vi "Lab Panel V5.24.1.vi"() -> ()   [LabVIEW 2013] (continued)
                          tunnel: [errorcluster {"status"=FALSE, "code"=0, "source"=""} ("error out") w884] -> w871
                          tunnel: w870 -> [_ w883]
                          tunnel: w869 -> [_ w882]
                          tunnel: w868 -> [_ w881]
                          tunnel: w867 -> [_ w880]
                          tunnel: w865 -> [_ w879]
                          frame False {
                            w877 = FALSE
                            n582 = local write "RUN LAB01-2"(w877) -> ()
                            n583 = local write "run lab01-2"(w877) -> ()
                          }
                          frame True {
                            n584 = stacked-sequence {
                              seq-local: [w890 _ _ _ _] -> [_ w914 _ _ _]
                              tunnel: w889 -> [w895 _ _ _ _]
                              tunnel: w888 -> [w892 _ _ _ _]
                              tunnel: w887 -> [w905 _ _ _ _]
                              tunnel: w886 -> [w898 _ _ _ _]
                              tunnel: w885 -> [w893 _ _ _ _]
                              tunnel: [_ w909 _ _ _] -> w884
                              tunnel: w883 -> [_ _ _ w936 _]
                              tunnel: w882 -> [_ _ _ w935 _]
                              tunnel: w881 -> [_ _ _ w934 _]
                              tunnel: w880 -> [_ _ _ _ _]
                              tunnel: w879 -> [_ _ _ _ w949]
                              frame #0 {
                                w891 = "\\"
                                n585 = local read "SET LAB01-2"() -> (w900:T5)
                                n586 = case shown="\"CYCLE TEST\"" w905 {
                                tunnel: ["L01-2-CHART TEST-" "L01-2-CYCLE TEST-" "L01-2-T-RISE TEST-"] -> w901
                                frame "CHART TEST", Default {
                                }
                                frame "CYCLE TEST" {
                                }
                                frame "T-RISE TEST" {
                                }
                                }
                                n587 = Unbundle(w900) -> ("DESCRIPTION"=w899:string)  [unwired: 4 out]
                                n588 = Concatenate Strings(w895, "\\", w893, w891, w892, w891) -> (w902:string)
                                n589 = String To Path(string=w902) -> (path=w904:path)
                                n590 = Concatenate Strings(w902, w901, w899, "-", w898, ".tdms") -> (w890:string)
                                n591 = Create Folder(path (use dialog)=w904) -> (error out=w903:errorcluster)  [unwired: 2 in, 2 out]
                                n592 = call <vilib>:"Clear Errors.vi"("error in (no error)"=w903) -> ()  [unwired: 6 in, 1 out]
                                n593 = global write "Global 1.vi" "LAB01-2 FILE"(w890) -> ()
                              }
                              frame #1 {
                                (unwired) FALSE
                                n594 = String To Path(string=w914) -> (path=w910:path)
                                n595 = TDMS Open(6:FALSE, 10:T21."create or replace" ("operation (0:open)"), 11:w910) -> (0:w909:errorcluster, 3:→"TDMS LAB01-2":refnum<k34>)  [unwired: 4 in]
                              }
                              frame #2 {
                                n596 = local read "SET LAB01-2"() -> (w920:T5)
                                n597 = local read "TDMS LAB01-2"() -> (w931:refnum<k34>)
                                n598 = Build Array("Testers Name", "Description", "Set Test Cycles", "T-Rise minutes", "T-Rise Deg C") -> (w921:string[])
                                n599 = Unbundle(w920) -> ("NAME"=w919:string, "DESCRIPTION"=w918:string, "CYCLES"=w917:dbl, "T-RISE mins"=w916:dbl, "T-RISE deg C"=w915:dbl)
                                n600 = Number To Decimal String(number=w917) -> (decimal integer string=w930:string)  [unwired: 1 in]
                                n601 = Number To Decimal String(number=w916) -> (decimal integer string=w929:string)  [unwired: 1 in]
                                n602 = Number To Decimal String(number=w915) -> (decimal integer string=w928:string)  [unwired: 1 in]
                                n603 = Build Array(w919, w918, w930, w929, w928) -> (w927:string[])
                                n604 = TDMS Set Properties(5:w927, 7:w921, 11:w931) -> ()  [unwired: 3 in, 4 out]
                              }
                              frame #3 {
                                n605 = local read "DISP LAB01-2"() -> (w933:T4)
                                n606 = Concatenate Strings("LAB01-2  ", w936) -> (w937:string)
                                n607 = Two Button Dialog(message=w937, 1:w934, 2:w935) -> (T button?=w939:bool)
                                n608 = case shown="True" w939 {
                                tunnel: w933 -> [w946 w947]
                                tunnel: [w946 w947] -> w943
                                tunnel: [w945 w948] -> w942
                                tunnel: [w944 w948] -> w941
                                frame False {
                                n609 = Unbundle(w946) -> ("CYCLE"=w945:dbl, "MINS"=w944:dbl)  [unwired: 1 out]
                                }
                                frame True {
                                w948 = 0.0
                                }
                                }
                                n610 = Bundle(cluster=w943, "CYCLE"=w942, "MINS"=w941, "STATUS"="RUN") -> (w932:T4)
                                n611 = local write "DISP LAB01-2"(w932) -> ()
                              }
                              frame #4 {
                                n612 = local read "TEMP START LAB01-2"() -> (w951:cluster{"TL":dbl, "TN":dbl})
                                n613 = Bundle(cluster=w951, "TL"=w949, "TN"=w949) -> (w950:cluster{"TL":dbl, "TN":dbl})
                                n614 = local write "TEMP START LAB01-2"(w950) -> ()
                              }
                            }
                          }
                        }
                      }
                    }
                  }
                }
              }
              event "RUN LAB02-1": Value Change {
                n615 = event-data() -> ("NewVal"=w957:bool)  [unwired: 1 in, 5 out]
                n616 = local read "SIG LAB02-1"() -> (w953:T2)
                n617 = case shown="True" w957 {
                  tunnel: w963 -> [_ w1001]
                  tunnel: w962 -> [_ w1000]
                  tunnel: w960 -> [w965 w999]
                  tunnel: w961 -> [_ w998]
                  tunnel: w959 -> [_ w997]
                  tunnel: [w964 w996] -> w958
                  tunnel: w956 -> [_ w995]
                  tunnel: w955 -> [_ w994]
                  tunnel: w954 -> [_ w993]
                  tunnel: w953 -> [_ w992]
                  tunnel: w952 -> [_ w991]
                  frame False {
                    # "stop test"
                    n618 = stacked-sequence {
                      tunnel: w965 -> [w974 _]
                      tunnel: [w966 _] -> w964
                      frame #0 {
                        n619 = local read "DISP LAB02-1"() -> (w973:T4)
                        n620 = Unbundle(w973) -> ("CYCLE"=w971:dbl, "MINS"=w972:dbl)  [unwired: 1 out]
                        n621 = case shown="\"CYCLE TEST\"" w974 {
                          tunnel: w972 -> [_ _ w981]
                          tunnel: w971 -> [w979 w980 _]
                          tunnel: [w979 w980 w981] -> w970
                          frame "CHART TEST", Default {
                          }
                          frame "CYCLE TEST" {
                          }
                          frame "T-RISE TEST" {
                          }
                        }
                        n622 = local read "TDMS LAB02-1"() -> (w978:refnum<k34>)
                        n623 = Build Array("STOPPED") -> (w975:string[])
                        n624 = Build Array(w970) -> (w969:dbl[])
                        n625 = TDMS Write(0:w978, 5:"TEST RESULT", 7:w975, 9:w969) -> (4:w967:refnum<k34>, 15:w968:errorcluster)  [unwired: 2 in, 2 out]
                        n626 = TDMS Close(8:w968, 11:w967) -> (0:w966:errorcluster)  [unwired: 1 out]
                      }
                      frame #1 {
                        n627 = local read "DISP LAB02-1"() -> (w985:T4)
                        n628 = stacked-sequence {
                          tunnel: "LAB02-1" -> [w987 w989]
                          frame #0 {
                            n629 = call "sub vi - defrag tdms v1.vi"("panel id"=w987) -> ("error out"=w986:errorcluster)  [unwired: 10 in]
                            n630 = local write "data file error"(w986) -> ()
                          }
                          frame #1 {
                            n631 = local write "RESULT LAB02-1"(FALSE) -> ()
                            n632 = call "Save data file (stop) v3.vi"("panel id"=w989) -> ("network file save error"=w988:errorcluster)  [unwired: 9 in, 1 out]
                            n633 = local write "data file error"(w988) -> ()
                          }
                        }
                        n634 = Bundle(cluster=w985, "STATUS"="STOP") -> (w983:T4)  [unwired: 2 in]
                        n635 = local write "DISP LAB02-1"(w983) -> ()
                      }
                    }
                  }
                  frame True {
                    n636 = stacked-sequence {
                      seq-local: [w1003 _] -> [_ w1007]
                      tunnel: w1001 -> [_ w1017]
                      tunnel: w1000 -> [_ w1016]
                      tunnel: w999 -> [_ w1015]
                      tunnel: w998 -> [_ w1014]
                      tunnel: w997 -> [_ w1013]
                      tunnel: [_ w1012] -> w996
                      tunnel: w995 -> [_ w1011]
                      tunnel: w994 -> [_ w1010]
                      tunnel: w993 -> [_ w1009]
                      tunnel: w992 -> [w1002 w1008]
                      tunnel: w991 -> [_ w1006]
                      frame #0 {
                        n637 = Unbundle(w1002) -> ("AMPS"=w1005:dbl)  [unwired: 4 out]
                        n638 = call "Check For Amps on v1.vi"("ID"="LAB02-1", "amps"=w1005) -> ("amps"=w1003:bool)  [unwired: 9 in]
                      }
                      frame #1 {
                        n639 = case shown="True" w1007 {
                          tunnel: w1017 -> [_ w1030]
                          tunnel: w1016 -> [_ w1029]
                          tunnel: w1015 -> [_ w1028]
                          tunnel: w1014 -> [_ w1027]
                          tunnel: w1013 -> [_ w1026]
                          tunnel: [errorcluster {"status"=FALSE, "code"=0, "source"=""} ("error out") w1025] -> w1012
                          tunnel: w1011 -> [_ w1024]
                          tunnel: w1010 -> [_ w1023]
                          tunnel: w1009 -> [_ w1022]
                          tunnel: w1008 -> [_ w1021]
                          tunnel: w1006 -> [_ w1020]
                          frame False {
                            w1019 = FALSE
                            n640 = local write "RUN LAB02-1"(w1019) -> ()
                            n641 = local write "run lab02-1"(w1019) -> ()
                          }
                          frame True {
                            n642 = stacked-sequence {
                              seq-local: [w1031 _ _ _ _] -> [_ w1055 _ _ _]
                              tunnel: w1030 -> [w1036 _ _ _ _]
                              tunnel: w1029 -> [w1033 _ _ _ _]
                              tunnel: w1028 -> [w1046 _ _ _ _]
                              tunnel: w1027 -> [w1039 _ _ _ _]
                              tunnel: w1026 -> [w1034 _ _ _ _]
                              tunnel: [_ w1050 _ _ _] -> w1025
                              tunnel: w1024 -> [_ _ _ w1076 _]
                              tunnel: w1023 -> [_ _ _ w1075 _]
                              tunnel: w1022 -> [_ _ _ w1074 _]
                              tunnel: w1021 -> [_ _ _ _ _]
                              tunnel: w1020 -> [_ _ _ _ w1090]
                              frame #0 {
                                w1032 = "\\"
                                n643 = local read "SET LAB02-1"() -> (w1041:T5)
                                n644 = case shown="\"CYCLE TEST\"" w1046 {
                                tunnel: ["L02-1-CHART TEST-" "L02-1-CYCLE TEST-" "L02-1-T-RISE TEST-"] -> w1042
                                frame "CHART TEST", Default {
                                }
                                frame "CYCLE TEST" {
                                }
                                frame "T-RISE TEST" {
                                }
                                }
                                n645 = Unbundle(w1041) -> ("DESCRIPTION"=w1040:string)  [unwired: 4 out]
                                n646 = Concatenate Strings(w1036, "\\", w1034, w1032, w1033, w1032) -> (w1043:string)
                                n647 = String To Path(string=w1043) -> (path=w1045:path)
                                n648 = Concatenate Strings(w1043, w1042, w1040, "-", w1039, ".tdms") -> (w1031:string)
                                n649 = Create Folder(path (use dialog)=w1045) -> (error out=w1044:errorcluster)  [unwired: 2 in, 2 out]
                                n650 = global write "Global 1.vi" "LAB02-1 FILE"(w1031) -> ()
                                n651 = call <vilib>:"Clear Errors.vi"("error in (no error)"=w1044) -> ()  [unwired: 6 in, 1 out]
                              }
                              frame #1 {
                                (unwired) FALSE
                                n652 = String To Path(string=w1055) -> (path=w1051:path)
                                n653 = TDMS Open(6:FALSE, 10:T21."create or replace" ("operation (0:open)"), 11:w1051) -> (0:w1050:errorcluster, 3:→"TDMS LAB02-1":refnum<k34>)  [unwired: 4 in]
                              }
                              frame #2 {
                                n654 = local read "SET LAB02-1"() -> (w1061:T5)
                                n655 = local read "TDMS LAB02-1"() -> (w1072:refnum<k34>)
                                n656 = Build Array("Testers Name", "Description", "Set Test Cycles", "T-Rise minutes", "T-Rise Deg C") -> (w1062:string[])
                                n657 = Unbundle(w1061) -> ("NAME"=w1060:string, "DESCRIPTION"=w1059:string, "CYCLES"=w1058:dbl, "T-RISE mins"=w1057:dbl, "T-RISE deg C"=w1056:dbl)
                                n658 = Number To Decimal String(number=w1058) -> (decimal integer string=w1071:string)  [unwired: 1 in]
                                n659 = Number To Decimal String(number=w1057) -> (decimal integer string=w1070:string)  [unwired: 1 in]
                                n660 = Number To Decimal String(number=w1056) -> (decimal integer string=w1069:string)  [unwired: 1 in]
                                n661 = Build Array(w1060, w1059, w1071, w1070, w1069) -> (w1068:string[])
                                n662 = TDMS Set Properties(5:w1068, 7:w1062, 11:w1072) -> ()  [unwired: 3 in, 4 out]
                              }
                              frame #3 {
                                n663 = local read "DISP LAB02-1"() -> (w1077:T4)
                                n664 = Concatenate Strings("LAB02-1  ", w1076) -> (w1078:string)
                                n665 = Two Button Dialog(message=w1078, 1:w1074, 2:w1075) -> (T button?=w1080:bool)
                                n666 = case shown="True" w1080 {
                                tunnel: w1077 -> [w1087 w1088]
                                tunnel: [w1087 w1088] -> w1084
                                tunnel: [w1086 w1089] -> w1083
                                tunnel: [w1085 w1089] -> w1082
                                frame False {
                                n667 = Unbundle(w1087) -> ("CYCLE"=w1086:dbl, "MINS"=w1085:dbl)  [unwired: 1 out]
                                }
                                frame True {
                                w1089 = 0.0
                                }
                                }
                                n668 = Bundle(cluster=w1084, "CYCLE"=w1083, "MINS"=w1082, "STATUS"="RUN") -> (w1073:T4)
                                n669 = local write "DISP LAB02-1"(w1073) -> ()
                              }
                              frame #4 {
                                n670 = local read "TEMP START LAB02-1"() -> (w1092:cluster{"TL":dbl, "TN":dbl})
                                n671 = Bundle(cluster=w1092, "TL"=w1090, "TN"=w1090) -> (w1091:cluster{"TL":dbl, "TN":dbl})
                                n672 = local write "TEMP START LAB02-1"(w1091) -> ()
                              }
                            }
                          }
                        }
                      }
                    }
                  }
                }
                n673 = local write "run lab02-1"(w957) -> ()
              }
              event "RUN LAB02-2": Value Change {
                n674 = event-data() -> ("NewVal"=w1097:bool)  [unwired: 1 in, 5 out]
                n675 = local write "run lab02-2"(w1097) -> ()
                n676 = case shown="True" w1097 {
                  tunnel: w1103 -> [_ w1141]
                  tunnel: w1102 -> [_ w1140]
                  tunnel: w1100 -> [w1105 w1139]
                  tunnel: w1101 -> [_ w1138]
                  tunnel: w1099 -> [_ w1137]
                  tunnel: [w1104 w1136] -> w1098
                  tunnel: w1096 -> [_ w1135]
                  tunnel: w1095 -> [_ w1134]
                  tunnel: w1094 -> [_ w1133]
                  tunnel: w1093 -> [_ w1131]
                  frame False {
                    # "stop test"
                    n677 = stacked-sequence {
                      tunnel: w1105 -> [w1114 _]
                      tunnel: [w1106 _] -> w1104
                      frame #0 {
                        n678 = local read "DISP LAB02-2"() -> (w1113:T4)
                        n679 = Unbundle(w1113) -> ("CYCLE"=w1111:dbl, "MINS"=w1112:dbl)  [unwired: 1 out]
                        n680 = case shown="\"CYCLE TEST\"" w1114 {
                          tunnel: w1112 -> [_ _ w1121]
                          tunnel: w1111 -> [w1119 w1120 _]
                          tunnel: [w1119 w1120 w1121] -> w1110
                          frame "CHART TEST", Default {
                          }
                          frame "CYCLE TEST" {
                          }
                          frame "T-RISE TEST" {
                          }
                        }
                        n681 = local read "TDMS LAB02-2"() -> (w1118:refnum<k34>)
                        n682 = Build Array("STOPPED") -> (w1115:string[])
                        n683 = Build Array(w1110) -> (w1109:dbl[])
                        n684 = TDMS Write(0:w1118, 5:"TEST RESULT", 7:w1115, 9:w1109) -> (4:w1107:refnum<k34>, 15:w1108:errorcluster)  [unwired: 2 in, 2 out]
                        n685 = TDMS Close(8:w1108, 11:w1107) -> (0:w1106:errorcluster)  [unwired: 1 out]
                      }
                      frame #1 {
                        n686 = local read "DISP LAB02-2"() -> (w1125:T4)
                        n687 = stacked-sequence {
                          tunnel: "LAB02-2" -> [w1127 w1129]
                          frame #0 {
                            n688 = call "sub vi - defrag tdms v1.vi"("panel id"=w1127) -> ("error out"=w1126:errorcluster)  [unwired: 10 in]
                            n689 = local write "data file error"(w1126) -> ()
                          }
                          frame #1 {
                            n690 = call "Save data file (stop) v3.vi"("panel id"=w1129) -> ("network file save error"=w1128:errorcluster)  [unwired: 9 in, 1 out]
                            n691 = local write "RESULT LAB02-2"(FALSE) -> ()
                            n692 = local write "data file error"(w1128) -> ()
                          }
                        }
                        n693 = Bundle(cluster=w1125, "STATUS"="STOP") -> (w1123:T4)  [unwired: 2 in]
                        n694 = local write "DISP LAB02-2"(w1123) -> ()
                      }
                    }
                  }
                  frame True {
                    n695 = local read "SIG LAB02-2"() -> (w1132:T2)
                    n696 = stacked-sequence {
                      seq-local: [w1143 _] -> [_ w1147]
                      tunnel: w1141 -> [_ w1157]
                      tunnel: w1140 -> [_ w1156]
                      tunnel: w1139 -> [_ w1155]
                      tunnel: w1138 -> [_ w1154]
                      tunnel: w1137 -> [_ w1153]
                      tunnel: [_ w1152] -> w1136
                      tunnel: w1135 -> [_ w1151]
                      tunnel: w1134 -> [_ w1150]
                      tunnel: w1133 -> [_ w1149]
                      tunnel: w1132 -> [w1142 w1148]
                      tunnel: w1131 -> [_ w1146]
                      frame #0 {
                        n697 = Unbundle(w1142) -> ("AMPS"=w1145:dbl)  [unwired: 4 out]
                        n698 = call "Check For Amps on v1.vi"("ID"="LAB02-2", "amps"=w1145) -> ("amps"=w1143:bool)  [unwired: 9 in]
                      }
                      frame #1 {
                        n699 = case shown="True" w1147 {
                          tunnel: w1157 -> [_ w1170]
                          tunnel: w1156 -> [_ w1169]
                          tunnel: w1155 -> [_ w1168]
                          tunnel: w1154 -> [_ w1167]
                          tunnel: w1153 -> [_ w1166]
                          tunnel: [errorcluster {"status"=FALSE, "code"=0, "source"=""} ("error out") w1165] -> w1152
                          tunnel: w1151 -> [_ w1164]
                          tunnel: w1150 -> [_ w1163]
                          tunnel: w1149 -> [_ w1162]
                          tunnel: w1148 -> [_ w1161]
                          tunnel: w1146 -> [_ w1160]
                          frame False {
                            w1158 = FALSE
                            n700 = local write "RUN LAB02-2"(w1158) -> ()
                            n701 = local write "run lab02-2"(w1158) -> ()
                          }
                          frame True {
                            n702 = stacked-sequence {
                              seq-local: [w1171 _ _ _ _] -> [_ w1195 _ _ _]
                              tunnel: w1170 -> [w1176 _ _ _ _]
                              tunnel: w1169 -> [w1173 _ _ _ _]
                              tunnel: w1168 -> [w1186 _ _ _ _]
                              tunnel: w1167 -> [w1179 _ _ _ _]
                              tunnel: w1166 -> [w1174 _ _ _ _]
                              tunnel: [_ w1190 _ _ _] -> w1165
                              tunnel: w1164 -> [_ _ _ w1216 _]
                              tunnel: w1163 -> [_ _ _ w1215 _]
                              tunnel: w1162 -> [_ _ _ w1214 _]
                              tunnel: w1161 -> [_ _ _ _ _]
                              tunnel: w1160 -> [_ _ _ _ w1230]
                              frame #0 {
                                w1172 = "\\"
                                n703 = local read "SET LAB02-2"() -> (w1181:T5)
                                n704 = case shown="\"CYCLE TEST\"" w1186 {
                                tunnel: ["L02-2-CHART TEST-" "L02-2-CYCLE TEST-" "L02-2-T-RISE TEST-"] -> w1182
                                frame "CHART TEST", Default {
                                }
                                frame "CYCLE TEST" {
                                }
                                frame "T-RISE TEST" {
                                }
                                }
                                n705 = Unbundle(w1181) -> ("DESCRIPTION"=w1180:string)  [unwired: 4 out]
                                n706 = Concatenate Strings(w1176, "\\", w1174, w1172, w1173, w1172) -> (w1183:string)
                                n707 = String To Path(string=w1183) -> (path=w1185:path)
                                n708 = Concatenate Strings(w1183, w1182, w1180, "-", w1179, ".tdms") -> (w1171:string)
                                n709 = Create Folder(path (use dialog)=w1185) -> (error out=w1184:errorcluster)  [unwired: 2 in, 2 out]
                                n710 = global write "Global 1.vi" "LAB02-2 FILE"(w1171) -> ()
                                n711 = call <vilib>:"Clear Errors.vi"("error in (no error)"=w1184) -> ()  [unwired: 6 in, 1 out]
                              }
                              frame #1 {
                                (unwired) FALSE
                                n712 = String To Path(string=w1195) -> (path=w1191:path)
                                n713 = TDMS Open(6:FALSE, 10:T21."create or replace" ("operation (0:open)"), 11:w1191) -> (0:w1190:errorcluster, 3:→"TDMS LAB02-2":refnum<k34>)  [unwired: 4 in]
                              }
                              frame #2 {
                                n714 = local read "SET LAB02-2"() -> (w1201:T5)
                                n715 = local read "TDMS LAB02-2"() -> (w1212:refnum<k34>)
                                n716 = Build Array("Testers Name", "Description", "Set Test Cycles", "T-Rise minutes", "T-Rise Deg C") -> (w1202:string[])
                                n717 = Unbundle(w1201) -> ("NAME"=w1200:string, "DESCRIPTION"=w1199:string, "CYCLES"=w1198:dbl, "T-RISE mins"=w1197:dbl, "T-RISE deg C"=w1196:dbl)
                                n718 = Number To Decimal String(number=w1198) -> (decimal integer string=w1211:string)  [unwired: 1 in]
                                n719 = Number To Decimal String(number=w1197) -> (decimal integer string=w1210:string)  [unwired: 1 in]
                                n720 = Number To Decimal String(number=w1196) -> (decimal integer string=w1209:string)  [unwired: 1 in]
                                n721 = Build Array(w1200, w1199, w1211, w1210, w1209) -> (w1208:string[])
                                n722 = TDMS Set Properties(5:w1208, 7:w1202, 11:w1212) -> ()  [unwired: 3 in, 4 out]
                              }
                              frame #3 {
                                n723 = local read "DISP LAB02-2"() -> (w1217:T4)
                                n724 = Concatenate Strings("LAB02-2  ", w1216) -> (w1218:string)
                                n725 = Two Button Dialog(message=w1218, 1:w1214, 2:w1215) -> (T button?=w1220:bool)
                                n726 = case shown="True" w1220 {
                                tunnel: w1217 -> [w1227 w1228]
                                tunnel: [w1227 w1228] -> w1224
                                tunnel: [w1226 w1229] -> w1223
                                tunnel: [w1225 w1229] -> w1222
                                frame False {
                                n727 = Unbundle(w1227) -> ("CYCLE"=w1226:dbl, "MINS"=w1225:dbl)  [unwired: 1 out]
                                }
                                frame True {
                                w1229 = 0.0
                                }
                                }
                                n728 = Bundle(cluster=w1224, "CYCLE"=w1223, "MINS"=w1222, "STATUS"="RUN") -> (w1213:T4)
                                n729 = local write "DISP LAB02-2"(w1213) -> ()
                              }
                              frame #4 {
                                n730 = local read "TEMP START LAB02-2"() -> (w1232:cluster{"TL":dbl, "TN":dbl})
                                n731 = Bundle(cluster=w1232, "TL"=w1230, "TN"=w1230) -> (w1231:cluster{"TL":dbl, "TN":dbl})
                                n732 = local write "TEMP START LAB02-2"(w1231) -> ()
                              }
                            }
                          }
                        }
                      }
                    }
                  }
                }
              }
              event "RUN LAB03-1": Value Change {
                n733 = event-data() -> ("NewVal"=w1237:bool)  [unwired: 1 in, 5 out]
                n734 = local write "run lab03-1"(w1237) -> ()
                n735 = case shown="True" w1237 {
                  tunnel: w1243 -> [_ w1281]
                  tunnel: w1242 -> [_ w1280]
                  tunnel: w1240 -> [w1245 w1279]
                  tunnel: w1241 -> [_ w1278]
                  tunnel: w1239 -> [_ w1277]
                  tunnel: [w1244 w1276] -> w1238
                  tunnel: w1236 -> [_ w1275]
                  tunnel: w1235 -> [_ w1274]
                  tunnel: w1234 -> [_ w1273]
                  tunnel: w1233 -> [_ w1271]
                  frame False {
                    # "stop test"
                    n736 = stacked-sequence {
                      tunnel: w1245 -> [w1254 _]
                      tunnel: [w1246 _] -> w1244
                      frame #0 {
                        n737 = local read "DISP LAB03-1"() -> (w1253:T4)
                        n738 = Unbundle(w1253) -> ("CYCLE"=w1251:dbl, "MINS"=w1252:dbl)  [unwired: 1 out]
                        n739 = case shown="\"CYCLE TEST\"" w1254 {
                          tunnel: w1252 -> [_ _ w1261]
                          tunnel: w1251 -> [w1259 w1260 _]
                          tunnel: [w1259 w1260 w1261] -> w1250
                          frame "CHART TEST", Default {
                          }
                          frame "CYCLE TEST" {
                          }
                          frame "T-RISE TEST" {
                          }
                        }
                        n740 = local read "TDMS LAB03-1"() -> (w1258:refnum<k34>)
                        n741 = Build Array("STOPPED") -> (w1255:string[])
                        n742 = Build Array(w1250) -> (w1249:dbl[])
                        n743 = TDMS Write(0:w1258, 5:"TEST RESULT", 7:w1255, 9:w1249) -> (4:w1247:refnum<k34>, 15:w1248:errorcluster)  [unwired: 2 in, 2 out]
                        n744 = TDMS Close(8:w1248, 11:w1247) -> (0:w1246:errorcluster)  [unwired: 1 out]
                      }
                      frame #1 {
                        n745 = local read "DISP LAB03-1"() -> (w1265:T4)
                        n746 = stacked-sequence {
                          tunnel: "LAB03-1" -> [w1267 w1269]
                          frame #0 {
                            n747 = call "sub vi - defrag tdms v1.vi"("panel id"=w1267) -> ("error out"=w1266:errorcluster)  [unwired: 10 in]
                            n748 = local write "data file error"(w1266) -> ()
                          }
                          frame #1 {
                            n749 = call "Save data file (stop) v3.vi"("panel id"=w1269) -> ("network file save error"=w1268:errorcluster)  [unwired: 9 in, 1 out]
                            n750 = local write "RESULT LAB03-1"(FALSE) -> ()
                            n751 = local write "data file error"(w1268) -> ()
                          }
                        }
                        n752 = Bundle(cluster=w1265, "STATUS"="STOP") -> (w1263:T4)  [unwired: 2 in]
                        n753 = local write "DISP LAB03-1"(w1263) -> ()
                      }
                    }
                  }
                  frame True {
                    n754 = local read "SIG LAB03-1"() -> (w1272:T2)
                    n755 = stacked-sequence {
                      seq-local: [w1283 _] -> [_ w1287]
                      tunnel: w1281 -> [_ w1297]
                      tunnel: w1280 -> [_ w1296]
                      tunnel: w1279 -> [_ w1295]
                      tunnel: w1278 -> [_ w1294]
                      tunnel: w1277 -> [_ w1293]
                      tunnel: [_ w1292] -> w1276
                      tunnel: w1275 -> [_ w1291]
                      tunnel: w1274 -> [_ w1290]
                      tunnel: w1273 -> [_ w1289]
                      tunnel: w1272 -> [w1282 w1288]
                      tunnel: w1271 -> [_ w1286]
                      frame #0 {
                        n756 = Unbundle(w1282) -> ("AMPS"=w1285:dbl)  [unwired: 4 out]
                        n757 = call "Check For Amps on v1.vi"("ID"="LAB03-1", "amps"=w1285) -> ("amps"=w1283:bool)  [unwired: 9 in]
                      }
                      frame #1 {
                        n758 = case shown="True" w1287 {
                          tunnel: w1297 -> [_ w1310]
                          tunnel: w1296 -> [_ w1309]
                          tunnel: w1295 -> [_ w1308]
                          tunnel: w1294 -> [_ w1307]
                          tunnel: w1293 -> [_ w1306]
                          tunnel: [errorcluster {"status"=FALSE, "code"=0, "source"=""} ("error out") w1305] -> w1292
                          tunnel: w1291 -> [_ w1304]
                          tunnel: w1290 -> [_ w1303]
                          tunnel: w1289 -> [_ w1302]
                          tunnel: w1288 -> [_ w1301]
                          tunnel: w1286 -> [_ w1300]
                          frame False {
                            w1298 = FALSE
                            n759 = local write "RUN LAB03-1"(w1298) -> ()
                            n760 = local write "run lab03-1"(w1298) -> ()
                          }
                          frame True {
                            n761 = stacked-sequence {
                              seq-local: [w1311 _ _ _ _] -> [_ w1335 _ _ _]
                              tunnel: w1310 -> [w1316 _ _ _ _]
                              tunnel: w1309 -> [w1313 _ _ _ _]
                              tunnel: w1308 -> [w1326 _ _ _ _]
                              tunnel: w1307 -> [w1319 _ _ _ _]
                              tunnel: w1306 -> [w1314 _ _ _ _]
                              tunnel: [_ w1330 _ _ _] -> w1305
                              tunnel: w1304 -> [_ _ _ w1355 _]
                              tunnel: w1303 -> [_ _ _ w1354 _]
                              tunnel: w1302 -> [_ _ _ w1353 _]
                              tunnel: w1301 -> [_ _ _ _ _]
                              tunnel: w1300 -> [_ _ _ _ w1370]
                              frame #0 {
                                w1312 = "\\"
                                n762 = local read "SET LAB03-1"() -> (w1321:T5)
                                n763 = case shown="\"T-RISE TEST\"" w1326 {
                                tunnel: ["L03-1-CHART TEST-" "L03-1-CYCLE TEST-" "L03-1-T-RISE TEST-"] -> w1322
                                frame "CHART TEST", Default {
                                }
                                frame "CYCLE TEST" {
                                }
                                frame "T-RISE TEST" {
                                }
                                }
                                n764 = Unbundle(w1321) -> ("DESCRIPTION"=w1320:string)  [unwired: 4 out]
                                n765 = Concatenate Strings(w1316, "\\", w1314, w1312, w1313, w1312) -> (w1323:string)
                                n766 = String To Path(string=w1323) -> (path=w1325:path)
                                n767 = Concatenate Strings(w1323, w1322, w1320, "-", w1319, ".tdms") -> (w1311:string)
                                n768 = Create Folder(path (use dialog)=w1325) -> (error out=w1324:errorcluster)  [unwired: 2 in, 2 out]
                                n769 = global write "Global 1.vi" "LAB03-1 FILE"(w1311) -> ()
                                n770 = call <vilib>:"Clear Errors.vi"("error in (no error)"=w1324) -> ()  [unwired: 6 in, 1 out]
                              }
                              frame #1 {
                                (unwired) FALSE
                                n771 = String To Path(string=w1335) -> (path=w1331:path)
                                n772 = TDMS Open(6:FALSE, 10:T21."create or replace" ("operation (0:open)"), 11:w1331) -> (0:w1330:errorcluster, 3:→"TDMS LAB03-1":refnum<k34>)  [unwired: 4 in]
                              }
                              frame #2 {
                                n773 = local read "SET LAB03-1"() -> (w1341:T5)
                                n774 = local read "TDMS LAB03-1"() -> (w1352:refnum<k34>)
                                n775 = Build Array("Testers Name", "Description", "Set Test Cycles", "T-Rise minutes", "T-Rise Deg C") -> (w1342:string[])
                                n776 = Unbundle(w1341) -> ("NAME"=w1340:string, "DESCRIPTION"=w1339:string, "CYCLES"=w1338:dbl, "T-RISE mins"=w1337:dbl, "T-RISE deg C"=w1336:dbl)
                                n777 = Number To Decimal String(number=w1338) -> (decimal integer string=w1351:string)  [unwired: 1 in]
                                n778 = Number To Decimal String(number=w1337) -> (decimal integer string=w1350:string)  [unwired: 1 in]
                                n779 = Number To Decimal String(number=w1336) -> (decimal integer string=w1349:string)  [unwired: 1 in]
                                n780 = Build Array(w1340, w1339, w1351, w1350, w1349) -> (w1348:string[])
                                n781 = TDMS Set Properties(5:w1348, 7:w1342, 11:w1352) -> ()  [unwired: 3 in, 4 out]
                              }
                              frame #3 {
                                n782 = local read "DISP LAB03-1"() -> (w1357:T4)
                                n783 = Concatenate Strings("LAB03-1  ", w1355) -> (w1358:string)
                                n784 = Two Button Dialog(message=w1358, 1:w1353, 2:w1354) -> (T button?=w1360:bool)
                                n785 = case shown="True" w1360 {
                                tunnel: w1357 -> [w1367 w1368]
                                tunnel: [w1367 w1368] -> w1364
                                tunnel: [w1366 w1369] -> w1363
                                tunnel: [w1365 w1369] -> w1362
                                frame False {
                                n786 = Unbundle(w1367) -> ("CYCLE"=w1366:dbl, "MINS"=w1365:dbl)  [unwired: 1 out]
                                }
                                frame True {
                                w1369 = 0.0
                                }
                                }
                                n787 = Bundle(cluster=w1364, "CYCLE"=w1363, "MINS"=w1362, "STATUS"="RUN") -> (w1356:T4)
                                n788 = local write "DISP LAB03-1"(w1356) -> ()
                              }
                              frame #4 {
                                n789 = local read "TEMP START LAB03-1"() -> (w1372:cluster{"TL":dbl, "TN":dbl})
                                n790 = Bundle(cluster=w1372, "TL"=w1370, "TN"=w1370) -> (w1371:cluster{"TL":dbl, "TN":dbl})
                                n791 = local write "TEMP START LAB03-1"(w1371) -> ()
                              }
                            }
                          }
                        }
                      }
                    }
                  }
                }
              }
              event "RUN LAB03-2": Value Change {
                n792 = event-data() -> ("NewVal"=w1377:bool)  [unwired: 1 in, 5 out]
                n793 = local write "run lab03-2"(w1377) -> ()
                n794 = case shown="True" w1377 {
                  tunnel: w1383 -> [_ w1421]
                  tunnel: w1382 -> [_ w1420]
                  tunnel: w1380 -> [w1385 w1419]
                  tunnel: w1381 -> [_ w1418]
                  tunnel: w1379 -> [_ w1417]
                  tunnel: [w1384 w1416] -> w1378
                  tunnel: w1376 -> [_ w1415]
                  tunnel: w1375 -> [_ w1414]
                  tunnel: w1374 -> [_ w1413]
                  tunnel: w1373 -> [_ w1411]
                  frame False {
                    # "stop test"
                    n795 = stacked-sequence {
                      tunnel: w1385 -> [w1394 _]
                      tunnel: [w1386 _] -> w1384
                      frame #0 {
                        n796 = local read "DISP LAB03-2"() -> (w1393:T4)
                        n797 = Unbundle(w1393) -> ("CYCLE"=w1391:dbl, "MINS"=w1392:dbl)  [unwired: 1 out]
                        n798 = case shown="\"CYCLE TEST\"" w1394 {
                          tunnel: w1392 -> [_ _ w1401]
                          tunnel: w1391 -> [w1399 w1400 _]
                          tunnel: [w1399 w1400 w1401] -> w1390
                          frame "CHART TEST", Default {
                          }
                          frame "CYCLE TEST" {
                          }
                          frame "T-RISE TEST" {
                          }
                        }
                        n799 = local read "TDMS LAB03-2"() -> (w1398:refnum<k34>)
                        n800 = Build Array("STOPPED") -> (w1395:string[])
                        n801 = Build Array(w1390) -> (w1389:dbl[])
                        n802 = TDMS Write(0:w1398, 5:"TEST RESULT", 7:w1395, 9:w1389) -> (4:w1387:refnum<k34>, 15:w1388:errorcluster)  [unwired: 2 in, 2 out]
                        n803 = TDMS Close(8:w1388, 11:w1387) -> (0:w1386:errorcluster)  [unwired: 1 out]
                      }
                      frame #1 {
                        n804 = local read "DISP LAB03-2"() -> (w1405:T4)
                        n805 = stacked-sequence {
                          tunnel: "LAB03-2" -> [w1407 w1409]
                          frame #0 {
                            n806 = call "sub vi - defrag tdms v1.vi"("panel id"=w1407) -> ("error out"=w1406:errorcluster)  [unwired: 10 in]
                            n807 = local write "data file error"(w1406) -> ()
                          }
                          frame #1 {
                            n808 = call "Save data file (stop) v3.vi"("panel id"=w1409) -> ("network file save error"=w1408:errorcluster)  [unwired: 9 in, 1 out]
                            n809 = local write "RESULT LAB03-2"(FALSE) -> ()
                            n810 = local write "data file error"(w1408) -> ()
                          }
                        }
                        n811 = Bundle(cluster=w1405, "STATUS"="STOP") -> (w1403:T4)  [unwired: 2 in]
                        n812 = local write "DISP LAB03-2"(w1403) -> ()
                      }
                    }
                  }
                  frame True {
                    n813 = local read "SIG LAB03-2"() -> (w1412:T2)
                    n814 = stacked-sequence {
                      seq-local: [w1423 _] -> [_ w1427]
                      tunnel: w1421 -> [_ w1437]
                      tunnel: w1420 -> [_ w1436]
                      tunnel: w1419 -> [_ w1435]
                      tunnel: w1418 -> [_ w1434]
                      tunnel: w1417 -> [_ w1433]
                      tunnel: [_ w1432] -> w1416
                      tunnel: w1415 -> [_ w1431]
                      tunnel: w1414 -> [_ w1430]
                      tunnel: w1413 -> [_ w1429]
                      tunnel: w1412 -> [w1422 w1428]
                      tunnel: w1411 -> [_ w1426]
                      frame #0 {
                        n815 = Unbundle(w1422) -> ("AMPS"=w1425:dbl)  [unwired: 4 out]
                        n816 = call "Check For Amps on v1.vi"("ID"="LAB03-2", "amps"=w1425) -> ("amps"=w1423:bool)  [unwired: 9 in]
                      }
                      frame #1 {
                        n817 = case shown="True" w1427 {
                          tunnel: w1437 -> [_ w1450]
                          tunnel: w1436 -> [_ w1449]
                          tunnel: w1435 -> [_ w1448]
                          tunnel: w1434 -> [_ w1447]
                          tunnel: w1433 -> [_ w1446]
                          tunnel: [errorcluster {"status"=FALSE, "code"=0, "source"=""} ("error out") w1445] -> w1432
                          tunnel: w1431 -> [_ w1444]
                          tunnel: w1430 -> [_ w1443]
                          tunnel: w1429 -> [_ w1442]
                          tunnel: w1428 -> [_ w1441]
                          tunnel: w1426 -> [_ w1440]
                          frame False {
                            w1438 = FALSE
                            n818 = local write "RUN LAB03-2"(w1438) -> ()
                            n819 = local write "run lab03-2"(w1438) -> ()
                          }
                          frame True {
                            n820 = stacked-sequence {
                              seq-local: [w1451 _ _ _ _] -> [_ w1475 _ _ _]
                              tunnel: w1450 -> [w1456 _ _ _ _]
                              tunnel: w1449 -> [w1453 _ _ _ _]
                              tunnel: w1448 -> [w1466 _ _ _ _]
                              tunnel: w1447 -> [w1459 _ _ _ _]
                              tunnel: w1446 -> [w1454 _ _ _ _]
                              tunnel: [_ w1470 _ _ _] -> w1445
                              tunnel: w1444 -> [_ _ _ w1496 _]
                              tunnel: w1443 -> [_ _ _ w1495 _]
                              tunnel: w1442 -> [_ _ _ w1494 _]
                              tunnel: w1441 -> [_ _ _ _ _]
                              tunnel: w1440 -> [_ _ _ _ w1510]
                              frame #0 {
                                w1452 = "\\"
                                n821 = local read "SET LAB03-2"() -> (w1461:T5)
                                n822 = case shown="\"T-RISE TEST\"" w1466 {
                                tunnel: ["L03-2-CHART TEST-" "L03-2-CYCLE TEST-" "L03-2-T-RISE TEST-"] -> w1462
                                frame "CHART TEST", Default {
                                }
                                frame "CYCLE TEST" {
                                }
                                frame "T-RISE TEST" {
                                }
                                }
                                n823 = Unbundle(w1461) -> ("DESCRIPTION"=w1460:string)  [unwired: 4 out]
                                n824 = Concatenate Strings(w1456, "\\", w1454, w1452, w1453, w1452) -> (w1463:string)
                                n825 = String To Path(string=w1463) -> (path=w1465:path)
                                n826 = Concatenate Strings(w1463, w1462, w1460, "-", w1459, ".tdms") -> (w1451:string)
                                n827 = Create Folder(path (use dialog)=w1465) -> (error out=w1464:errorcluster)  [unwired: 2 in, 2 out]
                                n828 = global write "Global 1.vi" "LAB03-2 FILE"(w1451) -> ()
                                n829 = call <vilib>:"Clear Errors.vi"("error in (no error)"=w1464) -> ()  [unwired: 6 in, 1 out]
                              }
                              frame #1 {
                                (unwired) FALSE
                                n830 = String To Path(string=w1475) -> (path=w1471:path)
                                n831 = TDMS Open(6:FALSE, 10:T21."create or replace" ("operation (0:open)"), 11:w1471) -> (0:w1470:errorcluster, 3:→"TDMS LAB03-2":refnum<k34>)  [unwired: 4 in]
                              }
                              frame #2 {
                                n832 = local read "SET LAB03-2"() -> (w1481:T5)
                                n833 = local read "TDMS LAB03-2"() -> (w1492:refnum<k34>)
                                n834 = Build Array("Testers Name", "Description", "Set Test Cycles", "T-Rise minutes", "T-Rise Deg C") -> (w1482:string[])
                                n835 = Unbundle(w1481) -> ("NAME"=w1480:string, "DESCRIPTION"=w1479:string, "CYCLES"=w1478:dbl, "T-RISE mins"=w1477:dbl, "T-RISE deg C"=w1476:dbl)
                                n836 = Number To Decimal String(number=w1478) -> (decimal integer string=w1491:string)  [unwired: 1 in]
                                n837 = Number To Decimal String(number=w1477) -> (decimal integer string=w1490:string)  [unwired: 1 in]
                                n838 = Number To Decimal String(number=w1476) -> (decimal integer string=w1489:string)  [unwired: 1 in]
                                n839 = Build Array(w1480, w1479, w1491, w1490, w1489) -> (w1488:string[])
                                n840 = TDMS Set Properties(5:w1488, 7:w1482, 11:w1492) -> ()  [unwired: 3 in, 4 out]
                              }
                              frame #3 {
                                n841 = local read "DISP LAB03-2"() -> (w1497:T4)
                                n842 = Concatenate Strings("LAB03-2  ", w1496) -> (w1498:string)
                                n843 = Two Button Dialog(message=w1498, 1:w1494, 2:w1495) -> (T button?=w1500:bool)
                                n844 = case shown="True" w1500 {
                                tunnel: w1497 -> [w1507 w1508]
                                tunnel: [w1507 w1508] -> w1504
                                tunnel: [w1506 w1509] -> w1503
                                tunnel: [w1505 w1509] -> w1502
                                frame False {
                                n845 = Unbundle(w1507) -> ("CYCLE"=w1506:dbl, "MINS"=w1505:dbl)  [unwired: 1 out]
                                }
                                frame True {
                                w1509 = 0.0
                                }
                                }
                                n846 = Bundle(cluster=w1504, "CYCLE"=w1503, "MINS"=w1502, "STATUS"="RUN") -> (w1493:T4)
                                n847 = local write "DISP LAB03-2"(w1493) -> ()
                              }
                              frame #4 {
                                n848 = local read "TEMP START LAB03-2"() -> (w1512:cluster{"TL":dbl, "TN":dbl})
                                n849 = Bundle(cluster=w1512, "TL"=w1510, "TN"=w1510) -> (w1511:cluster{"TL":dbl, "TN":dbl})
                                n850 = local write "TEMP START LAB03-2"(w1511) -> ()
                              }
                            }
                          }
                        }
                      }
                    }
                  }
                }
              }
              event "RUN LAB04-1": Value Change {
                n851 = event-data() -> ("NewVal"=w1517:bool)  [unwired: 1 in, 5 out]
